vi "Write to TDMS Log File (U8).vi"(6 "Data":u8[][](array[numeric]), 8 "error in (no error)":errorcluster, 9 "Channel Names in":string[](array[string]), 10 "Group Names in":string[](array[string]), 11 "TDMS Log File in":refnum<class "TDMS Log File.lvclass">) -> (0 "error out":errorcluster, 3 "TDMS Log File out":refnum<class "TDMS Log File.lvclass">)   [LabVIEW 2015, in "TDMS Log File.lvclass"]
uses:
  TDMS Log File.lvclass
  TDMS Log File.lvclass/TDMS Log File.ctl
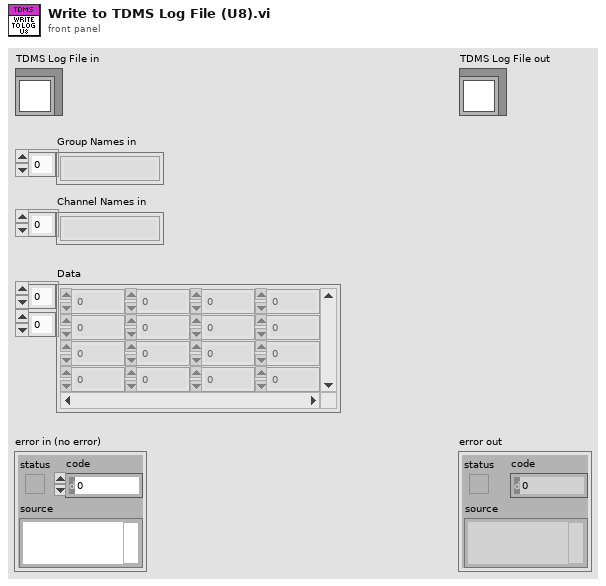
[diagram p1: front panel]
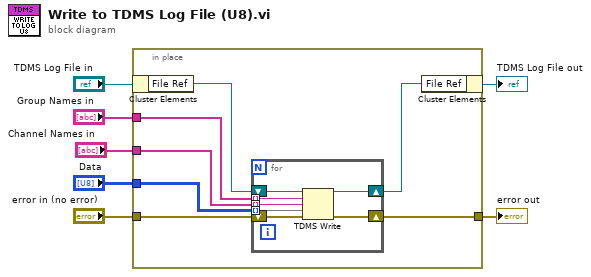
[diagram p0: block diagram]
diagram:
  n1 = in-place {
    in-place-border: "error in (no error)" -> [w14]
    in-place-border: [w12] -> w5
    in-place-border: "Data" -> [w8]
    in-place-border: "Group Names in" -> [w10]
    in-place-border: "Channel Names in" -> [w9]
    n2 = in-place-cluster #1("TDMS Log File in") -> ("File Ref"=w13:refnum<k34>)
    n3 = for {
      tunnel: w10 -> [w19] mode=indexing
      tunnel: w9 -> [w18] mode=indexing
      shift-right: [w16] -> w11
      shift-left: w13 -> [w20]
      tunnel: w8 -> [w17] mode=indexing
      shift-right: [w15] -> w12
      shift-left: w14 -> [w21]
      n4 = TDMS Write(0:w20, 5:w19, 7:w18, 9:w17, 11:w21) -> (4:w16:refnum<k34>, 15:w15:errorcluster)  [unwired: 1 in, 2 out]
    }
    n5 = in-place-cluster #1("File Ref"=w11) -> (→"TDMS Log File out":refnum<class "TDMS Log File.lvclass">)
  }
  "error out" <- w5
